vi "Get available devices.vi"(8 "error in (no error)":errorcluster, 11 "BMC in":refnum<class "BMC.lvclass">) -> (0 "error out":errorcluster, 3 "BMC out":refnum<class "BMC.lvclass">)   [LabVIEW 2012, in "BMC.lvclass"]
uses:
  BMC.lvclass
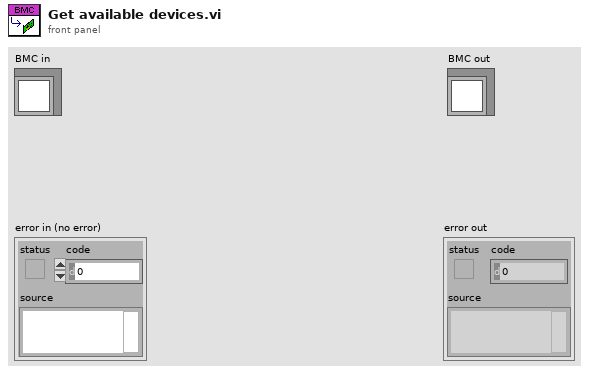
[diagram p1: front panel]
types:
  T1 = typedef "BMC.lvclass/CIUsbKub.IHostDrv.ctl" = refnum<k7>
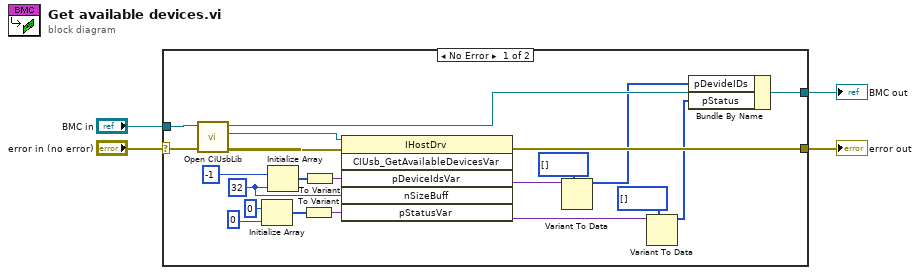
[diagram p0: block diagram]
diagram:
  n1 = case shown="No Error" "error in (no error)" {
    selector: "error in (no error)" -> [w10 w27]
    tunnel: [w15 w27] -> w3
    tunnel: [w12 w26] -> w1
    tunnel: "BMC in" -> [w8 w26]
    frame No Error {
      w19 = 32 ("dimension size")
      n2 = call-dynamic "Open CiUsbLib.vi"("error in (no error)"=w10, "BMC in"=w8) -> ("error out"=w9:errorcluster, "Automation Refnum"=w6:T1, "BMC out"=w7:refnum<class "BMC.lvclass">)  [unwired: 7 in]
      n3 = Initialize Array(i16 0 ("element"), 0 ("dimension size")) -> (w21:i16[])
      n4 = Initialize Array(i16 -1 ("element"), w19) -> (w18:i16[])
      n5 = To Variant(anything=w21) -> (Variant=w23:variant)
      n6 = To Variant(anything=w18) -> (Variant=w17:variant)
      n7 = invoke class="IHostDrv" method="CIUsb_GetAvailableDevicesVar"(reference=w6, error in=w9, "pDeviceIdsVar"=w17, "nSizeBuff"=w19, "pStatusVar"=w23) -> (error out=w15:errorcluster, "pDeviceIdsVar"=w24:variant, "pStatusVar"=w25:variant)  [unwired: 1 in, 3 out]
      n8 = Variant To Data(type=i32[] [] ("pDeviceIDs"), Variant=w24) -> (data=w5:i32[])  [unwired: 1 in, 1 out]
      n9 = Variant To Data(type=i32[] [] ("pStatus"), Variant=w25) -> (data=w11:i32[])  [unwired: 1 in, 1 out]
      n10 = Bundle By Name(cluster=w7, "pDevideIDs"=w5, "pStatus"=w11) -> (w12:refnum<class "BMC.lvclass">)
    }
    frame Error {
    }
  }
  "error out" <- w3
  "BMC out" <- w1
